vi "XCAN_Enable_&_Disable.vi"() -> ()   [LabVIEW 2016]
uses:
  <vilib>/Stratom, Inc/X-CAN for myRIO (API)/X-CAN Class/Type Definitions/CANFrame.ctl
  <vilib>/Stratom, Inc/X-Modules for myRIO/Type Defs/MXPChannel.ctl
  <vilib>/Stratom, Inc/X-CAN for myRIO (API)/X-CAN Class/Type Definitions/CAN_Speed.ctl
  <vilib>/myRIO/Common/Instrument Driver Framework/myRIO v1.0/UART/vis/myRIO v1.0 Close UART.vi
  <vilib>/myRIO/Common/Instrument Driver Framework/Utilities/vis/FPGA Ref Manager.vi
  <vilib>/myRIO/Common/Instrument Driver Framework/myRIO v1.0/myRIO v1.0 Reset FPGA.vi
  <vilib>/myRIO/Common/Instrument Driver Framework/myRIO v1.0/IRQ/vis/myRIO v1.0 IRQ Info FGV.vi
  <vilib>/myRIO/Common/Instrument Driver Framework/myRIO v1.0/IRQ/vis/myRIO v1.0 Timer IRQ Info FGV.vi
  <vilib>/myRIO/Common/Instrument Driver Framework/myRIO v1.0/IRQ/vis/myRIO v1.0 ISR Agent.vi
  <vilib>/Stratom, Inc/X-CAN for myRIO (API)/X-CAN Class/X-CAN.lvclass
  <vilib>/myRIO/Instrument Drivers/Utilities/Utilities.lvlib
panel:
  out "Disable_Mtr2":T1 {"payload" format="%x"; "timestamp" format="%<%I:%M:%S%8u %p\n%x>T"; "identifier" format="%x"}
  out "Enable_Mtr1":T1 {"payload" format="%x"; "timestamp" format="%<%I:%M:%S%8u %p\n%x>T"; "identifier" format="%x"}
  out "CAN Frame 8":T1 {"payload" format="%x"; "timestamp" format="%<%I:%M:%S%8u %p\n%x>T"; "identifier" format="%x"}
  out "Enable_Mtr2":T1 {"payload" format="%x"; "timestamp" format="%<%I:%M:%S%8u %p\n%x>T"; "identifier" format="%x"}
  out "CAN Frame 6":T1 {"payload" format="%x"; "timestamp" format="%<%I:%M:%S%8u %p\n%x>T"; "identifier" format="%x"}
  in  "Motor1(P)_______Motor2(D)":bool
  out "Disable_Mtr1":T1 {"payload" format="%x"; "timestamp" format="%<%I:%M:%S%8u %p\n%x>T"; "identifier" format="%x"}
  in  "Enable / Disable":bool
  # "Enable Status"
  # "Disable Status"
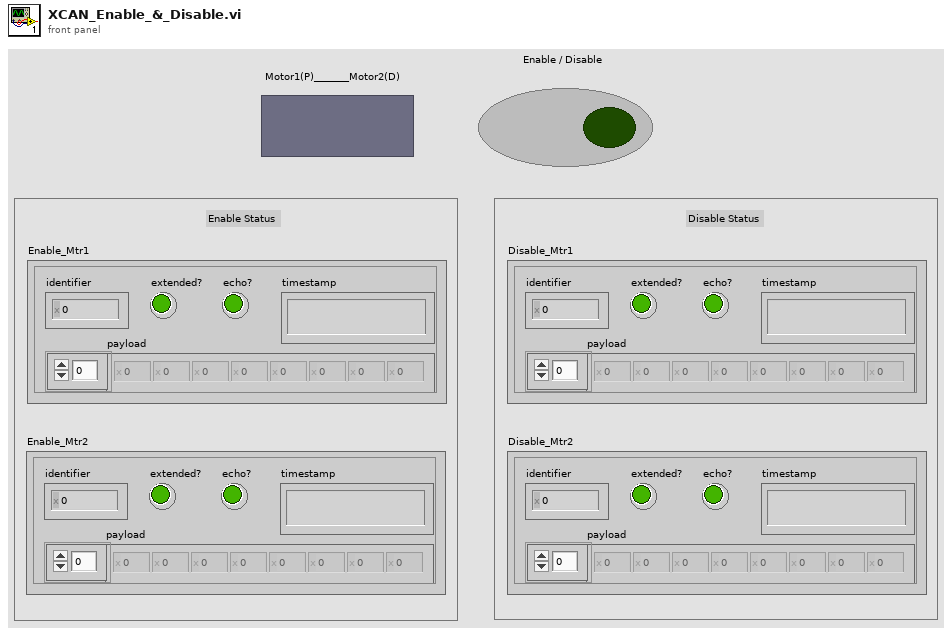
[diagram p1: front panel]
types:
  T1 = typedef "X-CAN.lvclass/CANFrame.ctl" = cluster{"identifier":u32, "extended?":bool, "echo?":bool, "payload":u8[], "timestamp":timestamp}
  T2 = typedef "X-CAN.lvclass/CAN_Speed.ctl" = u8
  T3 = typedef "MXPChannel.ctl" = enum16{"A/MXP", "B/MXP"}
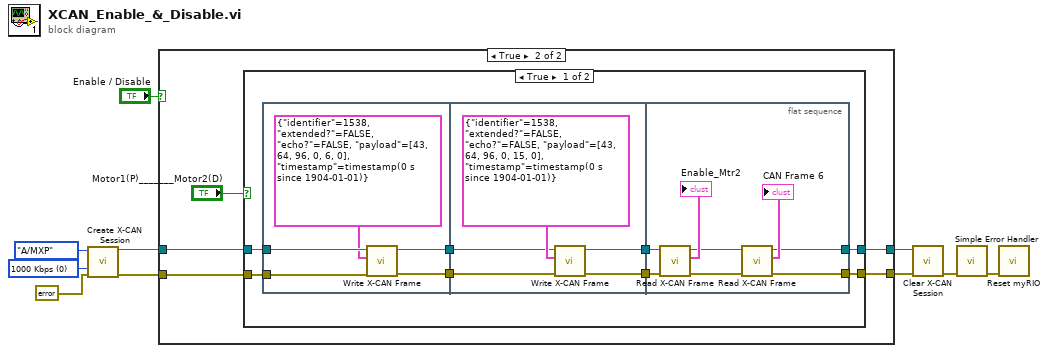
[diagram p0: block diagram]
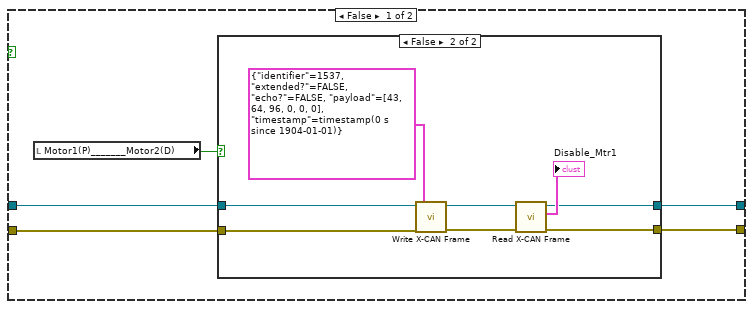
[diagram p2: hidden frame]
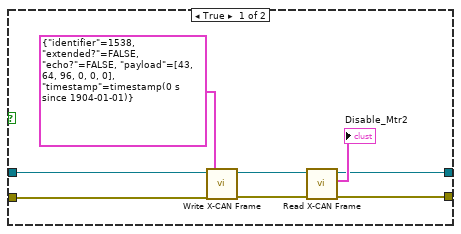
[diagram p3: hidden frame]
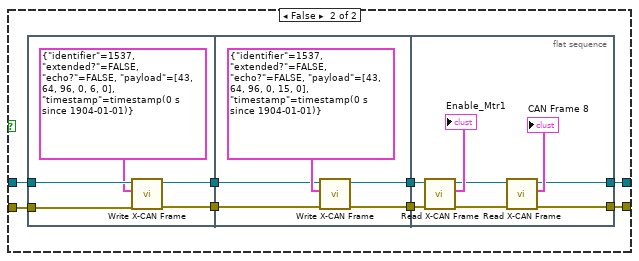
[diagram p4: hidden frame]
diagram:
  w7 = T2 0 items=["125 Kbps"=7, "250 Kbps"=3, "500 Kbps"=1, "1000 Kbps"=0, "95.238 Kbps"=6] ("CAN Speed [Kbps]")
  n1 = call <vilib>:"Create X-CAN Session.vi"("error in (no error)"=errorcluster {"status"=FALSE, "code"=0, "source"=""}, "CAN Speed [Kbps]"=w7, "MXP Channel"=MXPChannel."A/MXP") -> ("error out"=w5:errorcluster, "X-CAN Session out"=w4:refnum<class "X-CAN.lvclass">)  [unwired: 7 in]
  n2 = case shown="True" "Enable / Disable" {
    tunnel: [w13 w36] -> w1
    tunnel: [w12 w35] -> w2
    tunnel: w5 -> [w15 w34]
    tunnel: w4 -> [w14 w33]
    frame False {
      n3 = local read "Motor1(P)_______Motor2(D)"() -> (w11:bool)
      n4 = case shown="False" w11 {
        tunnel: w15 -> [w23 w31]
        tunnel: w14 -> [w22 w30]
        tunnel: [w18 w26] -> w13
        tunnel: [w16 w24] -> w12
        frame True {
          n5 = call <vilib>:"Write X-CAN Frame.vi"("error in"=w23, "CAN Frame"=T1 {"identifier"=1538, "extended?"=FALSE, "echo?"=FALSE, "payload"=[43, 64, 96, 0, 0, 0], "timestamp"=timestamp(0 s since 1904-01-01)}, "X-CAN Session in"=w22) -> ("error out"=w19:errorcluster, "X-CAN Session out"=w20:refnum<class "X-CAN.lvclass">)  [unwired: 7 in]
          n6 = call <vilib>:"Read X-CAN Frame.vi"("error in"=w19, "X-CAN Session in"=w20) -> ("error out"=w18:errorcluster, "CAN Frame"=→"Disable_Mtr2":T1, "X-CAN Session out"=w16:refnum<class "X-CAN.lvclass">)  [unwired: 7 in]
        }
        frame False {
          n7 = call <vilib>:"Write X-CAN Frame.vi"("error in"=w31, "CAN Frame"=T1 {"identifier"=1537, "extended?"=FALSE, "echo?"=FALSE, "payload"=[43, 64, 96, 0, 0, 0], "timestamp"=timestamp(0 s since 1904-01-01)}, "X-CAN Session in"=w30) -> ("error out"=w27:errorcluster, "X-CAN Session out"=w28:refnum<class "X-CAN.lvclass">)  [unwired: 7 in]
          n8 = call <vilib>:"Read X-CAN Frame.vi"("error in"=w27, "X-CAN Session in"=w28) -> ("error out"=w26:errorcluster, "CAN Frame"=→"Disable_Mtr1":T1, "X-CAN Session out"=w24:refnum<class "X-CAN.lvclass">)  [unwired: 7 in]
        }
      }
    }
    frame True {
      n9 = case shown="True" "Motor1(P)_______Motor2(D)" {
        tunnel: [w40 w66] -> w36
        tunnel: [w39 w65] -> w35
        tunnel: w34 -> [w38 w64]
        tunnel: w33 -> [w37 w63]
        frame True {
          n10 = flat-sequence {
            tunnel: w38 -> [w47]
            tunnel: w37 -> [w46]
            tunnel: [w49] -> w44
            tunnel: [w48] -> w43
            tunnel: w44 -> [w52]
            tunnel: w43 -> [w53]
            tunnel: [w51] -> w42
            tunnel: [w50] -> w41
            tunnel: [w55] -> w39
            tunnel: [w60] -> w40
            tunnel: w42 -> [w62]
            tunnel: w41 -> [w59]
            frame #0 {
              n11 = call <vilib>:"Write X-CAN Frame.vi"("error in"=w47, "CAN Frame"=T1 {"identifier"=1538, "extended?"=FALSE, "echo?"=FALSE, "payload"=[43, 64, 96, 0, 6, 0], "timestamp"=timestamp(0 s since 1904-01-01)}, "X-CAN Session in"=w46) -> ("error out"=w49:errorcluster, "X-CAN Session out"=w48:refnum<class "X-CAN.lvclass">)  [unwired: 7 in]
            }
            frame #1 {
              n12 = call <vilib>:"Write X-CAN Frame.vi"("error in"=w52, "CAN Frame"=T1 {"identifier"=1538, "extended?"=FALSE, "echo?"=FALSE, "payload"=[43, 64, 96, 0, 15, 0], "timestamp"=timestamp(0 s since 1904-01-01)}, "X-CAN Session in"=w53) -> ("error out"=w51:errorcluster, "X-CAN Session out"=w50:refnum<class "X-CAN.lvclass">)  [unwired: 7 in]
            }
            frame #2 {
              n13 = call <vilib>:"Read X-CAN Frame.vi"("error in"=w62, "X-CAN Session in"=w59) -> ("error out"=w61:errorcluster, "CAN Frame"=→"Enable_Mtr2":T1, "X-CAN Session out"=w56:refnum<class "X-CAN.lvclass">)  [unwired: 7 in]
              n14 = call <vilib>:"Read X-CAN Frame.vi"("error in"=w61, "X-CAN Session in"=w56) -> ("error out"=w60:errorcluster, "CAN Frame"=→"CAN Frame 6":T1, "X-CAN Session out"=w55:refnum<class "X-CAN.lvclass">)  [unwired: 7 in]
            }
          }
        }
        frame False {
          n15 = flat-sequence {
            tunnel: w64 -> [w73]
            tunnel: w63 -> [w72]
            tunnel: [w75] -> w70
            tunnel: [w74] -> w69
            tunnel: w70 -> [w78]
            tunnel: w69 -> [w79]
            tunnel: [w77] -> w68
            tunnel: [w76] -> w67
            tunnel: [w81] -> w65
            tunnel: [w86] -> w66
            tunnel: w68 -> [w88]
            tunnel: w67 -> [w85]
            frame #0 {
              n16 = call <vilib>:"Write X-CAN Frame.vi"("error in"=w73, "CAN Frame"=T1 {"identifier"=1537, "extended?"=FALSE, "echo?"=FALSE, "payload"=[43, 64, 96, 0, 6, 0], "timestamp"=timestamp(0 s since 1904-01-01)}, "X-CAN Session in"=w72) -> ("error out"=w75:errorcluster, "X-CAN Session out"=w74:refnum<class "X-CAN.lvclass">)  [unwired: 7 in]
            }
            frame #1 {
              n17 = call <vilib>:"Write X-CAN Frame.vi"("error in"=w78, "CAN Frame"=T1 {"identifier"=1537, "extended?"=FALSE, "echo?"=FALSE, "payload"=[43, 64, 96, 0, 15, 0], "timestamp"=timestamp(0 s since 1904-01-01)}, "X-CAN Session in"=w79) -> ("error out"=w77:errorcluster, "X-CAN Session out"=w76:refnum<class "X-CAN.lvclass">)  [unwired: 7 in]
            }
            frame #2 {
              n18 = call <vilib>:"Read X-CAN Frame.vi"("error in"=w88, "X-CAN Session in"=w85) -> ("error out"=w87:errorcluster, "CAN Frame"=→"Enable_Mtr1":T1, "X-CAN Session out"=w82:refnum<class "X-CAN.lvclass">)  [unwired: 7 in]
              n19 = call <vilib>:"Read X-CAN Frame.vi"("error in"=w87, "X-CAN Session in"=w82) -> ("error out"=w86:errorcluster, "CAN Frame"=→"CAN Frame 8":T1, "X-CAN Session out"=w81:refnum<class "X-CAN.lvclass">)  [unwired: 7 in]
            }
          }
        }
      }
    }
  }
  n20 = call <vilib>:"Clear X-CAN Session.vi"("error in (no error)"=w1, "X-CAN Session in"=w2) -> ("error out"=w10:errorcluster)  [unwired: 9 in]
  n21 = call <vilib>:"Simple Error Handler.vi"("error in (no error)"=w10) -> ("error out"=w9:errorcluster)  [unwired: 4 in, 4 out]
  n22 = call <vilib>:"Reset myRIO.vi"("error in (no error)"=w9) -> ()  [unwired: 10 in, 1 out]
